vi "Observe Data.vi"(6 "Time Stamp":timestamp, 8 "error in (no error)":errorcluster, 9 "Value":variant, 10 "Datum Name":string, 11 "ObservingModel In":refnum<class "ObservingModel.lvclass">) -> (0 "error out":errorcluster, 3 "ObservingModel Out":refnum<class "ObservingModel.lvclass">)   [LabVIEW 2017, in "ObservingModel.lvclass"]
doc: "<License>\nCopyright © 2017 Composed Systems, LLC | All rights reserved\nwww.composed.io\n\nAuthor: Ethan Stern <ethan.stern@composed.io>\n\nThis software is provided \"AS IS\" WITHOUT WARRANTIES, either express or implied, AND IS FOR EDUCATIONAL PURPOSES ONLY.\n</License>"
uses:
  ObservingModel.lvclass
  ObservingModel.lvclass/ObservingModel.ctl
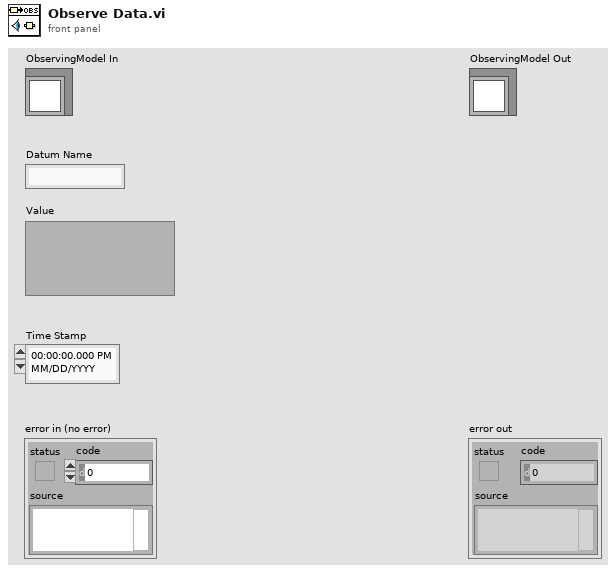
[diagram p1: front panel]
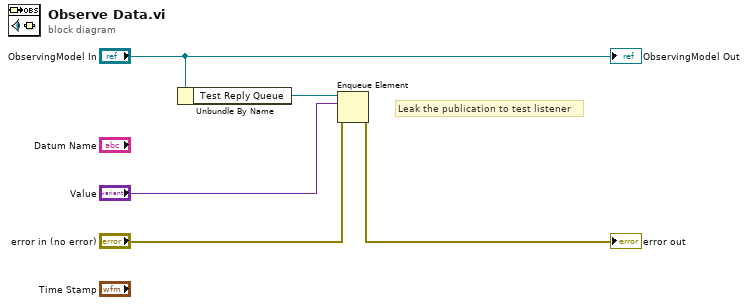
[diagram p0: block diagram]
diagram:
  # "Leak the publication to test listener"
  n1 = Unbundle By Name("ObservingModel In") -> ("Test Reply Queue"=w4:refnum<queue>)
  n2 = Enqueue Element(queue=w4, element="Value", error in (no error)="error in (no error)") -> (error out=→"error out":errorcluster)  [unwired: 1 in, 2 out]
  "ObservingModel Out" <- "ObservingModel In"
